vi "spreed_sheet_example.vi"() -> ()   [LabVIEW 2016]
uses:
  <vilib>/Utility/file.llb/Write Delimited Spreadsheet (DBL).vi
  <vilib>/Utility/file.llb/Read Delimited Spreadsheet (DBL).vi
panel:
  out "all rows":dbl[][](array[numeric])
  in  "file path (dialog if empty)":path
  out "Array":dbl[][](array[numeric])
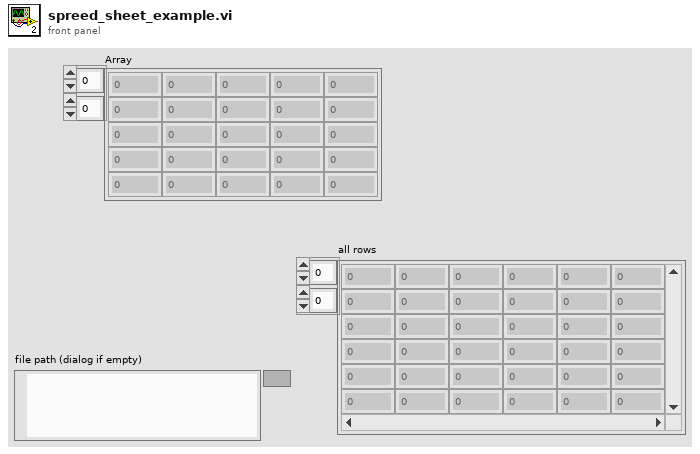
[diagram p1: front panel]
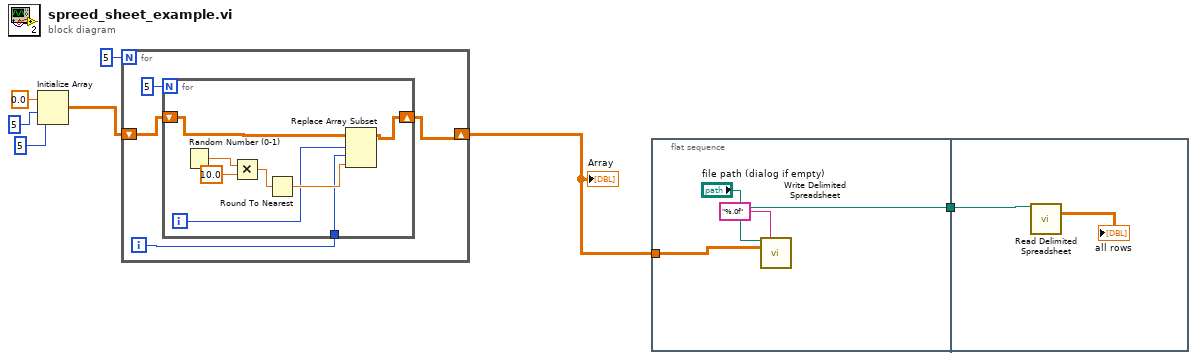
[diagram p0: block diagram]
diagram:
  n1 = Initialize Array(0.0 ("element"), 5 ("dimension size"), 5 ("dimension size")) -> (w4:dbl[][])
  n2 = for {
    N: 5 -> [_]
    shift-right: [w10] -> w2
    shift-left: w4 -> [w11]
    i -> [w8]
    n3 = for {
      N: 5 -> [_]
      shift-right: [w14] -> w10
      shift-left: w11 -> [w15]
      tunnel: w8 -> [w12]
      i -> [w13]
      n4 = Random Number (0-1)() -> (number: 0 to 1=w19:dbl)
      n5 = Multiply(x=w19, y=10.0) -> (x*y=w17:dbl)
      n6 = Round To Nearest(number=w17) -> (nearest integer value=w16:dbl)
      n7 = Replace Array Subset(array=w15, new element=w16, index (row)=w13, index (col)=w12) -> (w14:dbl[][])
    }
  }
  "Array" <- w2
  n8 = flat-sequence {
    tunnel: w2 -> [w22]
    tunnel: ["file path (dialog if empty)"] -> w1
    tunnel: w1 -> [w24]
    frame #0 {
      n9 = call-poly <vilib>:"Write Delimited Spreadsheet.vi"("file path (dialog if empty)"="file path (dialog if empty)", "format (%.3f)"="%.0f", "2D data"=w22) -> ()  [unwired: 11 in, 2 out]
    }
    frame #1 {
      n10 = call-poly <vilib>:"Read Delimited Spreadsheet.vi"("file path (dialog if empty)"=w24) -> ("all rows"=→"all rows":dbl[][])  [unwired: 9 in, 5 out]
    }
  }
